vi "Ejercicio_3_2.vi"() -> ()   [LabVIEW 2020]
panel:
  out "max value":i32
  out "element":i32
  out "Nivel Fluidos":dynamicdata(graph)
  out "Array 2":dbl[](array[numeric])
  out "Array":dbl[](array[numeric])
  out "Agua":dbl(slide) scale=0.0..50.0
  out "Aceite":dbl(slide) scale=0.0..10.0
  out "Numeric":i32
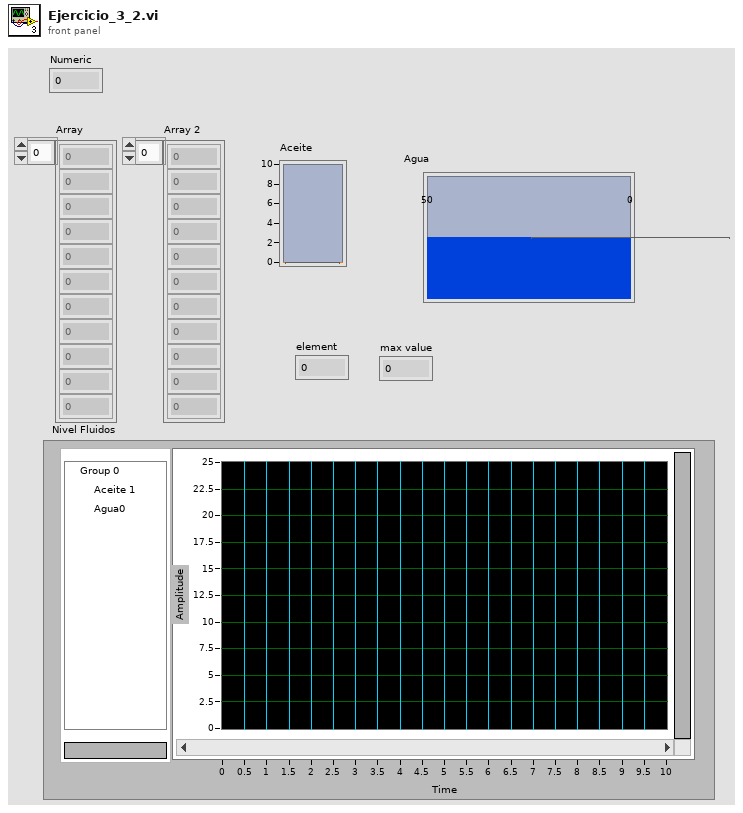
[diagram p1: front panel]
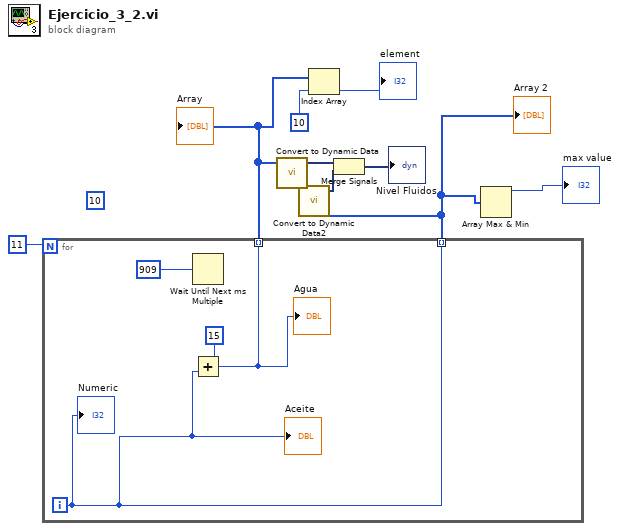
[diagram p0: block diagram]
diagram:
  (unwired) 10
  n1 = for {
    N: 11 -> [_]
    tunnel: [w11] -> w5 mode=indexing
    tunnel: [w10] -> w2 mode=indexing
    i -> [w10]
    n2 = Wait Until Next ms Multiple(millisecond multiple=909) -> ()  [unwired: 1 out]
    n3 = Add(x=15, y=w10) -> (x+y=w11:i32)
    "Agua" <- w11
    "Aceite" <- w10
    "Numeric" <- w10
  }
  "Array" <- w5
  "Array 2" <- w2
  n4 = call "Convert to Dynamic Data"("Array"=w5) -> ("Dynamic Data Type"=w8:dynamicdata)  [unwired: 3 in]
  n5 = call "Convert to Dynamic Data2"("Array"=w2) -> ("Dynamic Data Type"=w7:dynamicdata)  [unwired: 3 in]
  n6 = Index Array(array=w5, index=10) -> (element=→"element":i32)
  n7 = Merge Signals(w8, w7) -> (→"Nivel Fluidos":dynamicdata)
  n8 = Array Max & Min(array=w2) -> (max value=→"max value":i32)  [unwired: 3 out]
